vi "_word.GetBookmarks.vi"(8 "error in (no error)":errorcluster, 11 "Automation Refnum in":refnum<k7>) -> (0 "error out":errorcluster, 3 "Array":string[](array[string]))   [LabVIEW 2018, in "WordReportGeneration.lvlib"]
uses:
  WordReportGeneration.lvlib
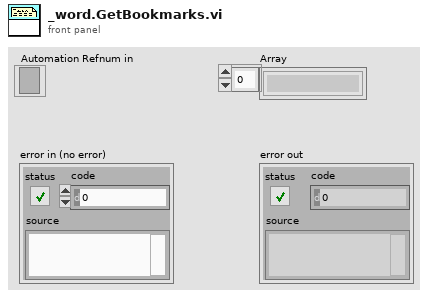
[diagram p1: front panel]
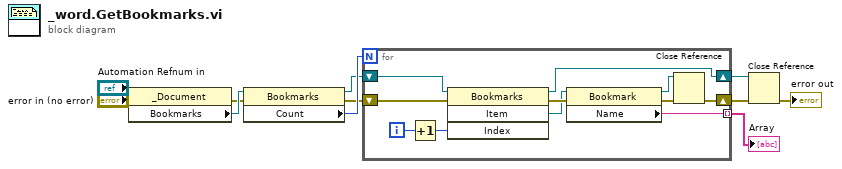
[diagram p0: block diagram]
diagram:
  n1 = property class="_Document"(reference="Automation Refnum in", error in="error in (no error)") -> (error out=w7:errorcluster, "Bookmarks"=w11:refnum<k7>)  [unwired: 1 out]
  n2 = property class="Bookmarks"(reference=w11, error in=w7) -> (reference out=w8:refnum<k7>, error out=w9:errorcluster, "Count"=w10:i32)
  n3 = for {
    N: w10 -> [_]
    tunnel: [w18] -> w1 mode=indexing
    shift-right: [w15] -> w6
    shift-left: w9 -> [w17]
    shift-right: [w12] -> w5
    shift-left: w8 -> [w16]
    i -> [w21]
    n4 = Increment(x=w21) -> (x+1=w20:i32)
    n5 = invoke class="Bookmarks" method="Item"(reference=w16, error in=w17, "Index"=w20) -> (reference out=w12:refnum<k7>, error out=w22:errorcluster, "Item"=w19:refnum<k7>)  [unwired: 1 in, 1 out]
    n6 = property class="Bookmark"(reference=w19, error in=w22) -> (reference out=w13:refnum<k7>, error out=w14:errorcluster, "Name"=w18:string)
    n7 = Close Reference(reference=w13, error in (no error)=w14) -> (error out=w15:errorcluster)
  }
  "Array" <- w1
  n8 = Close Reference(reference=w5, error in (no error)=w6) -> (error out=→"error out":errorcluster)
